vi "Create All Message Queues.vi"(8 "error in (no error)":errorcluster, 10 "DUT":string, 11 "This VI":refnum<vi>) -> (0 "error out":errorcluster, 3 "Message Queues out":T1)   [LabVIEW 2024, in "PCANusb_DTU.lvlib" / "PCAN Message Queue.lvlib"]
doc: "This VI creates and initializes all the message queues for your application. If your application requires more than one message queue, right-click the \"Message Queues\" constant above and select Open Type Def. Add the new Message Queue(s) to the type definition, then initialize them in this VI."
uses:
  PCAN Message Queue.lvlib
  All Message Queues.ctl
  Enqueue Message (Single).vi
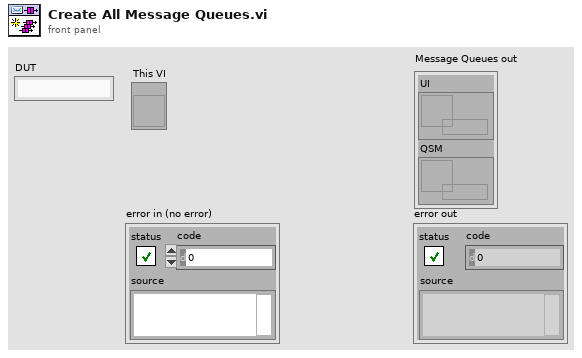
[diagram p1: front panel]
types:
  T1 = typedef "PCANusb_DTU.lvlib/PCAN Message Queue.lvlib/All Message Queues.ctl" = cluster{"UI":refnum<queue>, "QSM":refnum<queue>}
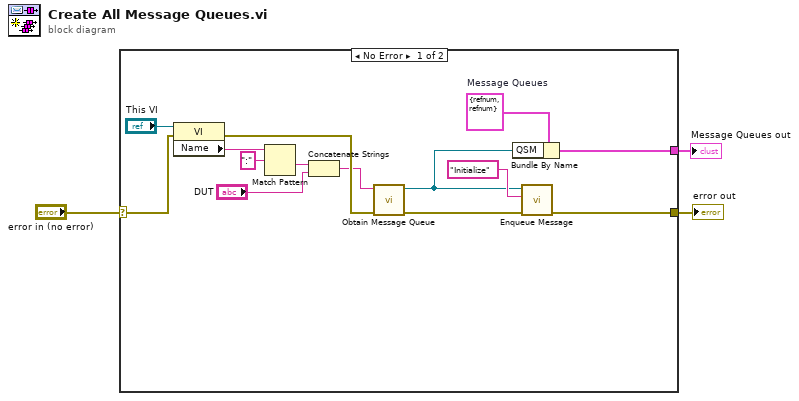
[diagram p0: block diagram]
diagram:
  n1 = case shown="No Error" "error in (no error)" {
    selector: "error in (no error)" -> [w9 w18]
    tunnel: [w17 w18] -> w3
    tunnel: [w15 _] -> w2
    frame No Error {
      w16 = T1 {"UI"=refnum, "QSM"=refnum}  # Message Queues
      n2 = property class="VI"(reference="This VI", error in=w9) -> (error out=w8:errorcluster, "Name"=w11:string)  [unwired: 1 out]
      n3 = Match Pattern(string=w11, regular expression=":") -> (after substring=w7:string)  [unwired: 1 in, 3 out]
      n4 = Concatenate Strings(w7, "DUT") -> (w5:string)
      n5 = call "Obtain Message Queue.vi"("error in (no error)"=w8, "Queue Name"=w5) -> ("error out"=w14:errorcluster, "Message Queue"=w12:refnum<queue>)  [unwired: 8 in]
      n6 = Bundle By Name(cluster=w16, "QSM"=w12) -> (w15:T1)
      n7 = call-poly "Enqueue Message.vi"("error in (no error)"=w14, "Message"="Initialize", "Message Queue"=w12) -> ("error out"=w17:errorcluster)  [unwired: 7 in, 1 out]
    }
    frame Error {
    }
  }
  "Message Queues out" <- w2
  "error out" <- w3
